vi "ABB Test Instruments.vi"() -> ()   [LabVIEW 2017]
uses:
  ABB global.vi
panel:
  in  "Instrument List":string[][](table)
  in  "Exit":bool
  # "Test Instruments"
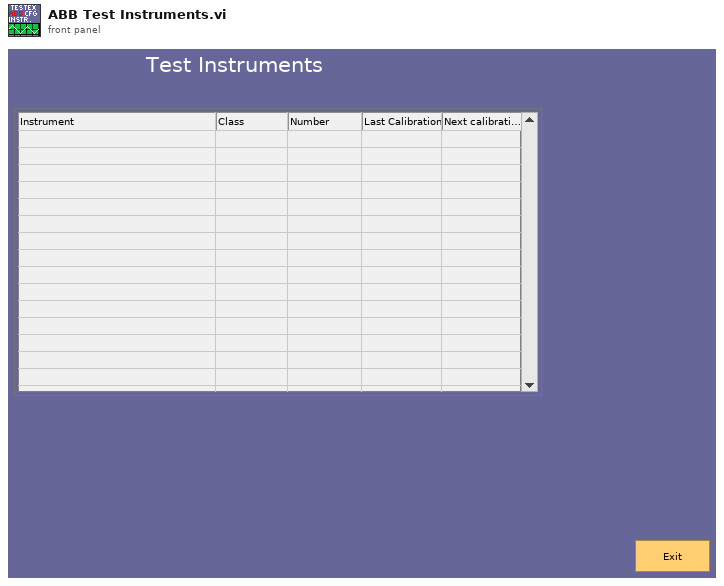
[diagram p1: front panel]
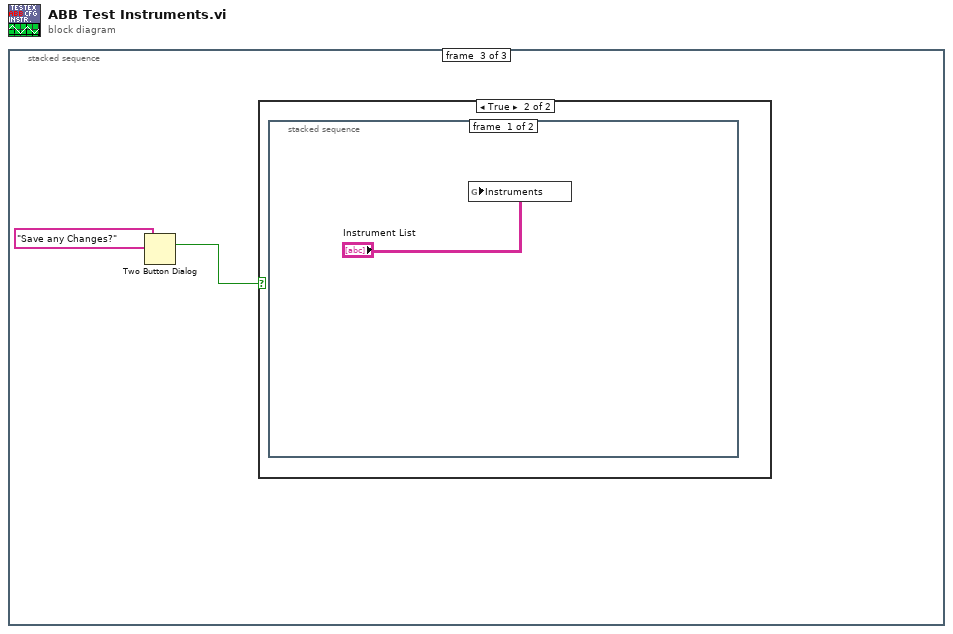
[diagram p0: block diagram]
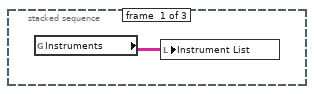
[diagram p2: hidden frame]
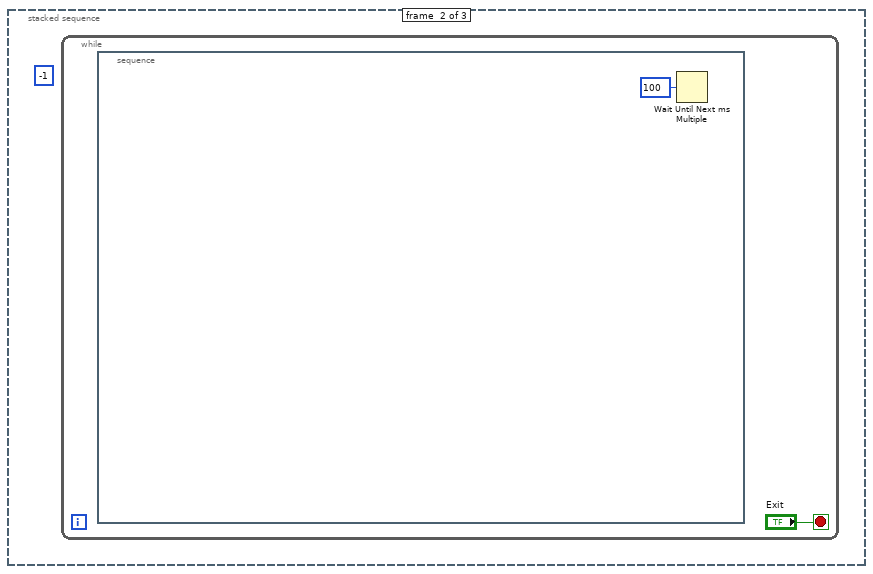
[diagram p3: hidden frame]
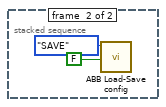
[diagram p5: hidden frame]
diagram:
  n1 = stacked-sequence {
    frame #0 {
      n2 = global read "ABB global.vi" "Instruments"() -> (w1:string[][])
      n3 = local write "Instrument List"(w1) -> ()
    }
    frame #1 {
      (unwired) -1 ("Number Values")
      n4 = while {
        stop <- "Exit" stop-if-true
        n5 = stacked-sequence {
          frame #0 {
            n6 = Wait Until Next ms Multiple(millisecond multiple=u32 100) -> ()  [unwired: 1 out]
          }
        }
      }
    }
    frame #2 {
      n7 = Two Button Dialog(message="Save any Changes?") -> (T button?=w5:bool)  [unwired: 2 in]
      n8 = case shown="True" w5 {
        frame False {
        }
        frame True {
          n9 = stacked-sequence {
            frame #0 {
              n10 = global write "ABB global.vi" "Instruments"("Instrument List") -> ()
            }
            frame #1 {
              n11 = call "ABB Load-Save config.vi"("confirm save"=FALSE, "Mode"=enum16{"LOAD", "SAVE"}."SAVE") -> ()  [unwired: 10 in]
            }
          }
        }
      }
    }
  }
